vi "Set.vi"(10 "Entity ID":T1, 11 "ID in":refnum<class "ID.lvclass">) -> (3 "ID out":refnum<class "ID.lvclass">)   [LabVIEW 2022 SP3, in "Conditum.lvlib" / "Columns.lvlib" / "ID.lvclass"]
uses:
  ID.lvclass
  Entity ID.ctl
  ID.lvclass/ID.ctl
  Conditum.lvlib
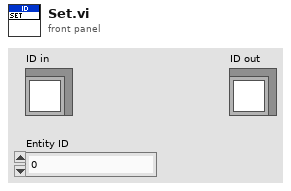
[diagram p1: front panel]
types:
  T1 = typedef "Conditum.lvlib/Entity ID.ctl" = i64
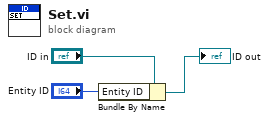
[diagram p0: block diagram]
diagram:
  n1 = Bundle By Name(cluster="ID in", "Entity ID"="Entity ID") -> (→"ID out":refnum<class "ID.lvclass">)
